vi "RP Read Temperature VISA.vi"(8 "Error In":errorcluster, 11 "VISA resource":refnum<visa-resource-name>) -> (0 "error out":errorcluster, 2 "Thermometer":dbl(slide)=48.847186279148 scale=0.0..100.0, 3 "VISA resource out":refnum<visa-resource-name>)   [LabVIEW 2019]
uses:
  RP Command.ctl
  RP Write Command VISA.vi
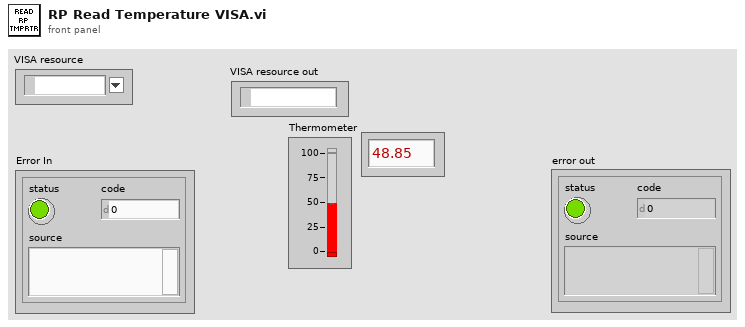
[diagram p1: front panel]
types:
  T1 = enum16{"big-endian, network order", "native, host order", "little-endian"}
  T2 = typedef "RP Command.ctl" = enum16{"Reset", "Read IDN", "Stop server", "Get status", "Get temperature", "Connect client", "Arm", "Software trigger", "Get whole buffer", "Get chunk", "System call", "Get config", "Set config", "Recieve data", "Recieve Calibartion", "Transmit data"}
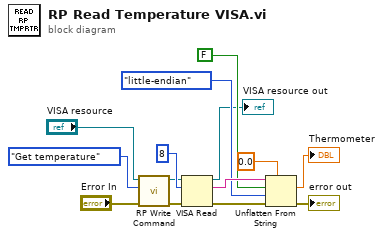
[diagram p0: block diagram]
diagram:
  n1 = call-poly "RP Write Command.vi"("Error In"="Error In", "Command number"=RP_Command."Get temperature", "VISA resource"="VISA resource") -> ("Error Out"=w7:errorcluster, "VISA resource out"=w6:refnum<visa-resource-name>)  [unwired: 6 in, 1 out]
  n2 = VISA Read(VISA resource name=w6, byte count=u32 8 ("bytes to read"), error in (no error)=w7) -> (VISA resource name out=→"VISA resource out":refnum<visa-resource-name>, read buffer=w13:string, error out=w11:errorcluster)  [unwired: 1 out]
  n3 = Unflatten From String(type=0.0, binary string=w13, data includes array or string size? (T)=FALSE, byte order (0:big-endian, network order)=T1."little-endian", error in (no error)=w11) -> (value=→"Thermometer":dbl, error out=→"error out":errorcluster)  [unwired: 1 out]
